vi "Piezo Message Loop.vi"(8 "error in (no error)":errorcluster, 10 "Data Notifiers":T1, 11 "Message Queues":T2) -> (0 "error out":errorcluster)   [LabVIEW 2013, in "Piezo.lvlib"]
uses:
  Piezo.lvlib
  support/Message Queue/All Message Queues.ctl
  support/Message Queue/Message Cluster.ctl
  support/Data Notifiers/All Data Notifiers.ctl
  Acquisition/APD Notifier Cluster.ctl
  Piezo display.ctl
  XY/XY Display.ctl
  Capacitive/Capacitive Signal Cluster.ctl
  Feedback/Error Signal.ctl
  Piezo State.ctl
  Untitled Project 3 Andrea/piezo new/Hardware Configuration Piezo out.ctl
  support/Message Queue/Enqueue Message (Single).vi
  <vilib>/Utility/error.llb/Error Cluster From Error Code.vi
  <vilib>/ErrorRing/Error Ring.xnode
  support/Message Queue/Message Queue.lvlib
  Acquisition/Acquisition.lvlib
  XY/XY.lvlib
  support/Data Notifiers/Data Notifiers.lvlib
  Capacitive/Capacitive.lvlib
  Feedback/Feedback.lvlib
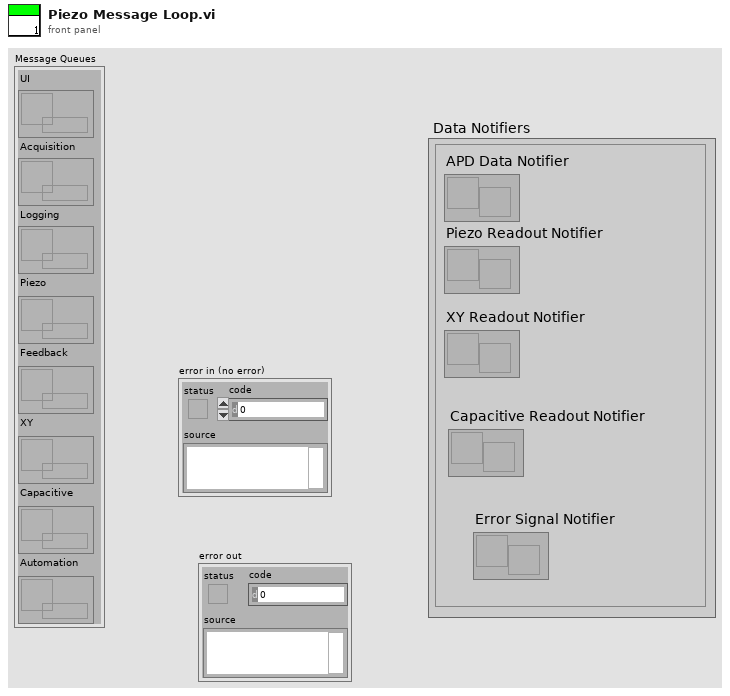
[diagram p1: front panel]
types:
  T1 = typedef "Data Notifiers.lvlib/All Data Notifiers.ctl" = cluster{"APD Data Notifier":refnum<notifier>, "Piezo Readout Notifier":refnum<notifier>, "XY Readout Notifier":refnum<notifier>, "Capacitive Readout Notifier":refnum<notifier>, "Error Signal Notifier":refnum<notifier>}
  T2 = typedef "Message Queue.lvlib/All Message Queues.ctl" = cluster{"UI":refnum<queue>, "Acquisition":refnum<queue>, "Logging":refnum<queue>, "Piezo":refnum<queue>, "Feedback":refnum<queue>, "XY":refnum<queue>, "Capacitive":refnum<queue>, "Automation":refnum<queue>}
  T3 = typedef "Hardware Configuration Piezo out.ctl" = cluster{"physical channels":tag, "MAX   VOLTAGE":dbl, "MIN   VOLTAGE":dbl}
  T4 = typedef "Piezo.lvlib/Piezo State.ctl" = enum16{"Idle", "Acquiring"}
  T5 = typedef "Acquisition.lvlib/APD Notifier Cluster.ctl" = cluster{"data":dbl[][], "t0":i32}
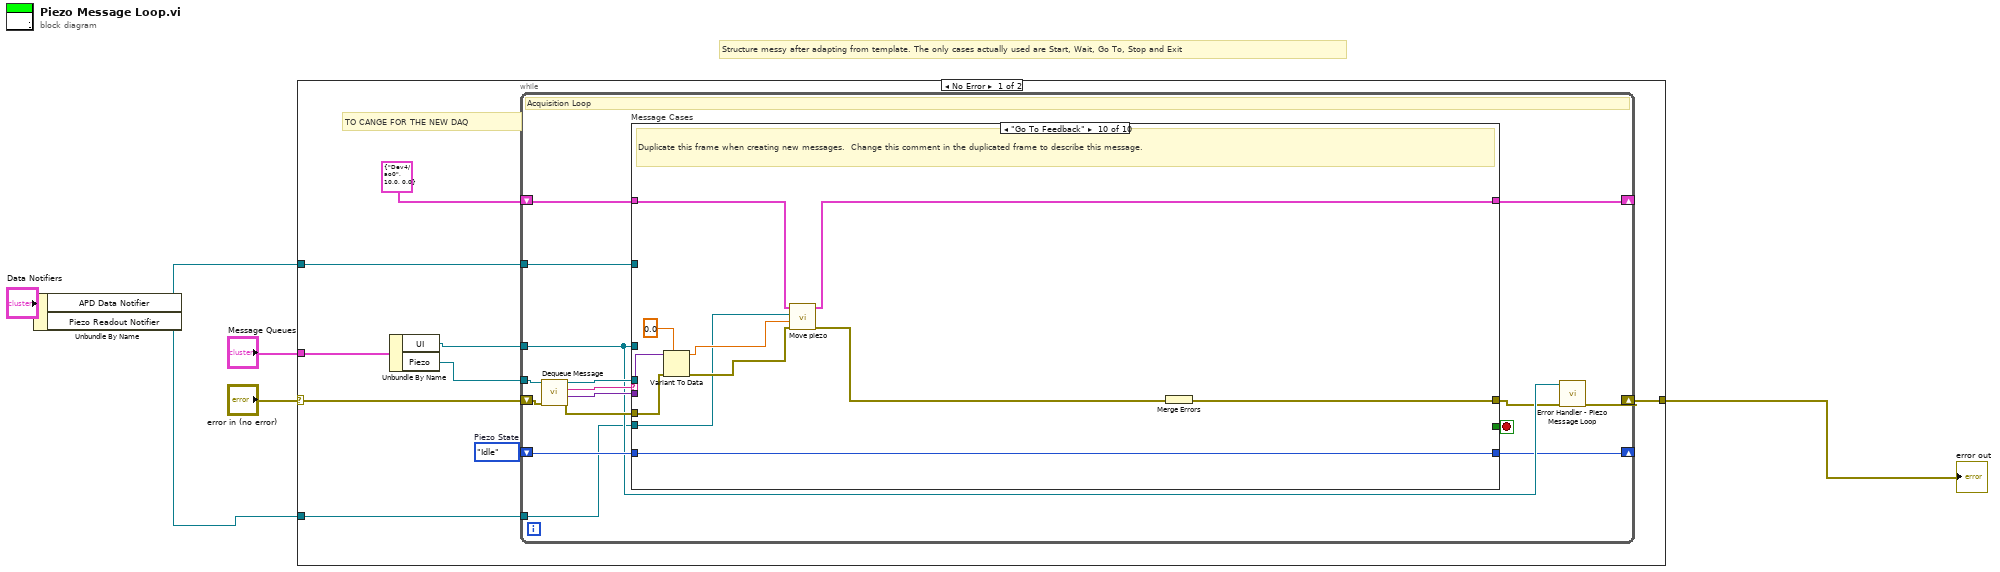
[diagram p0: block diagram]
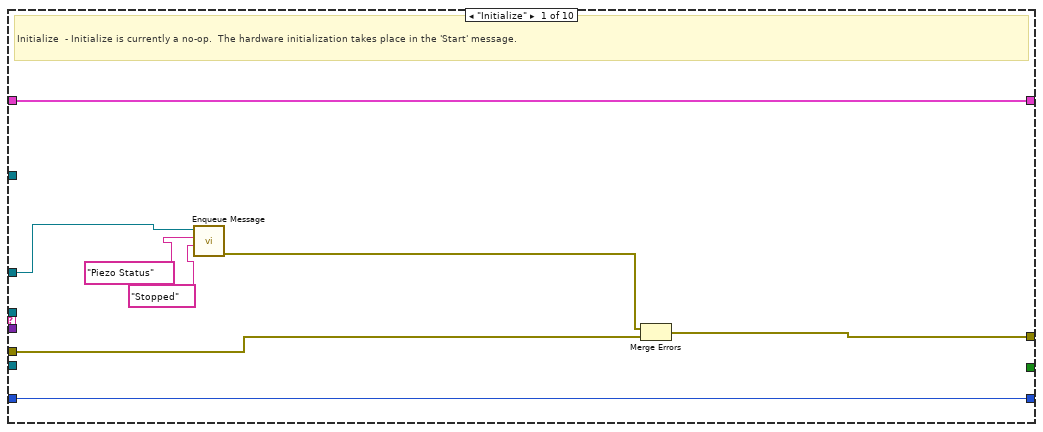
[diagram p2: hidden frame]
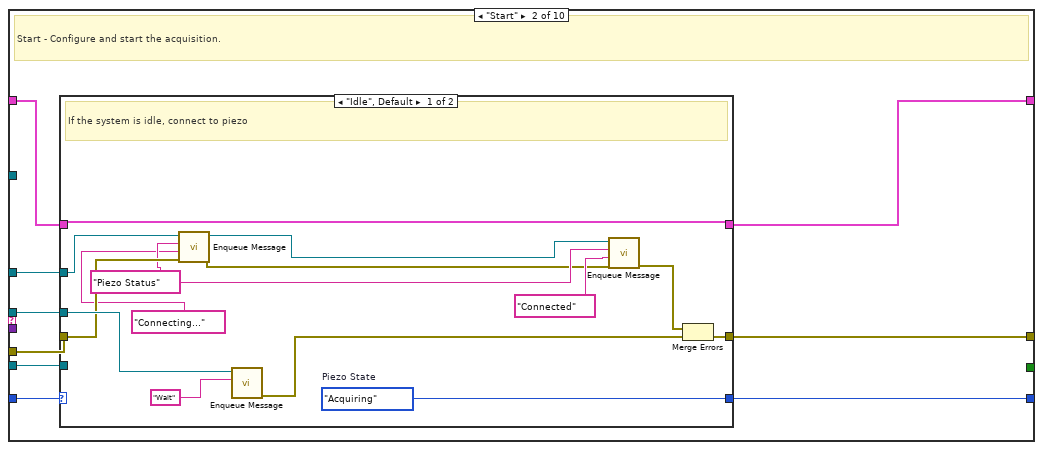
[diagram p3: hidden frame]
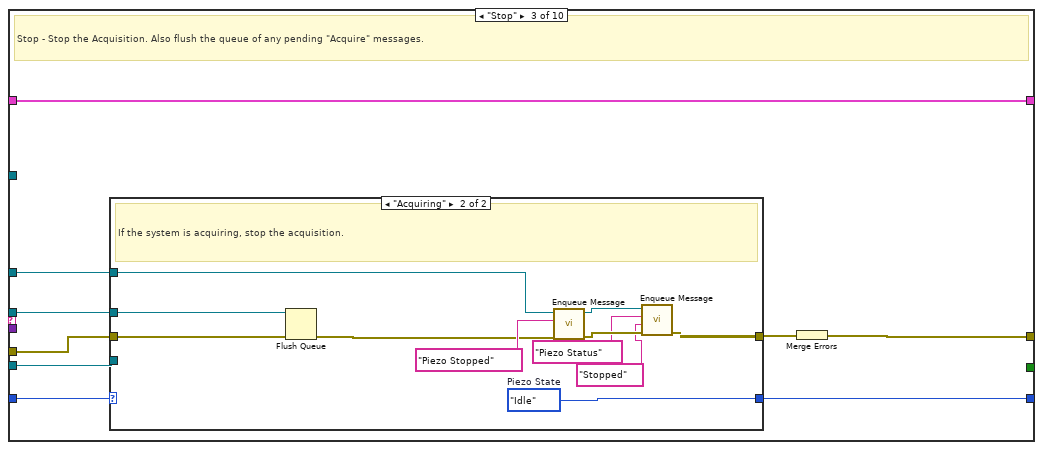
[diagram p5: hidden frame]
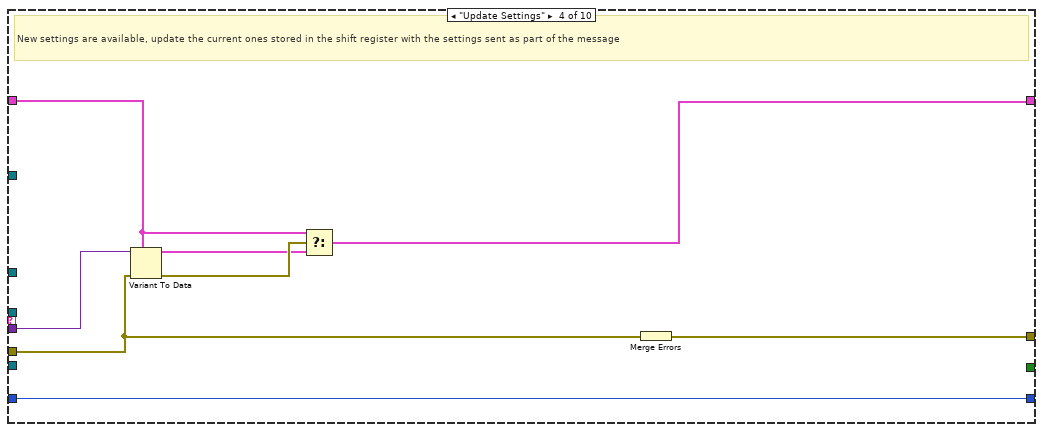
[diagram p7: hidden frame]
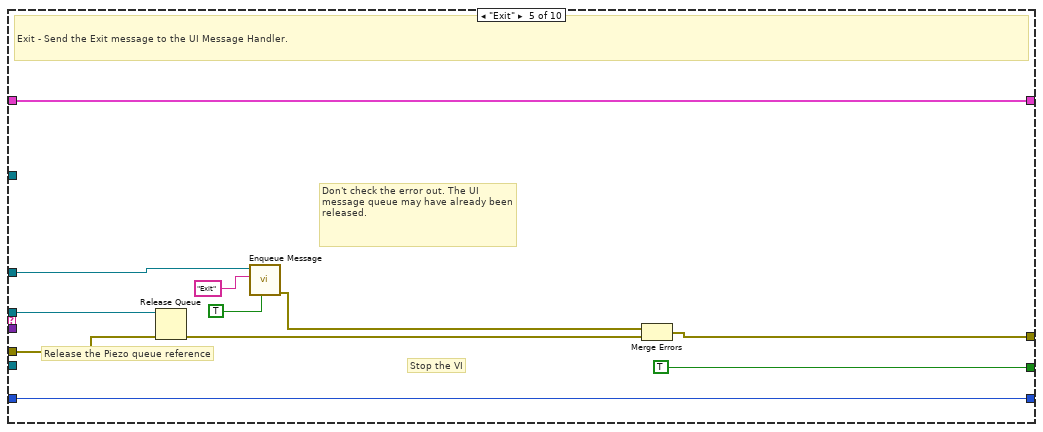
[diagram p8: hidden frame]
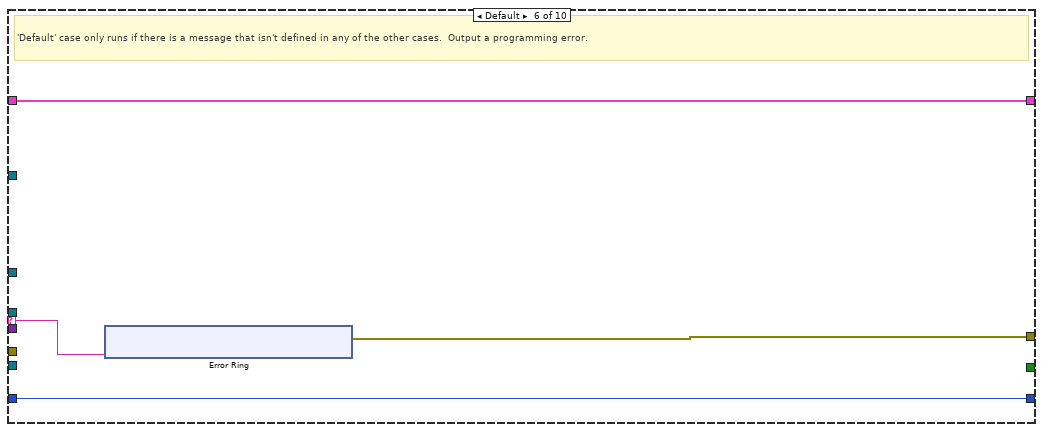
[diagram p9: hidden frame]
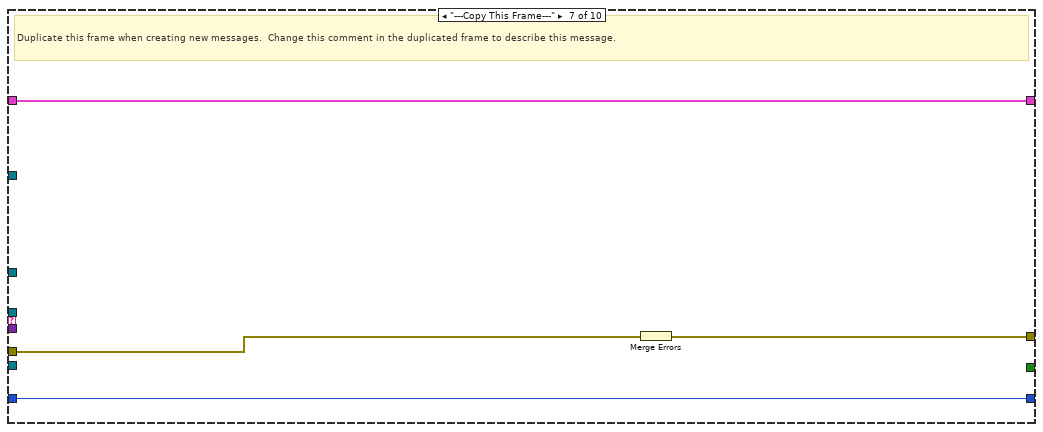
[diagram p10: hidden frame]
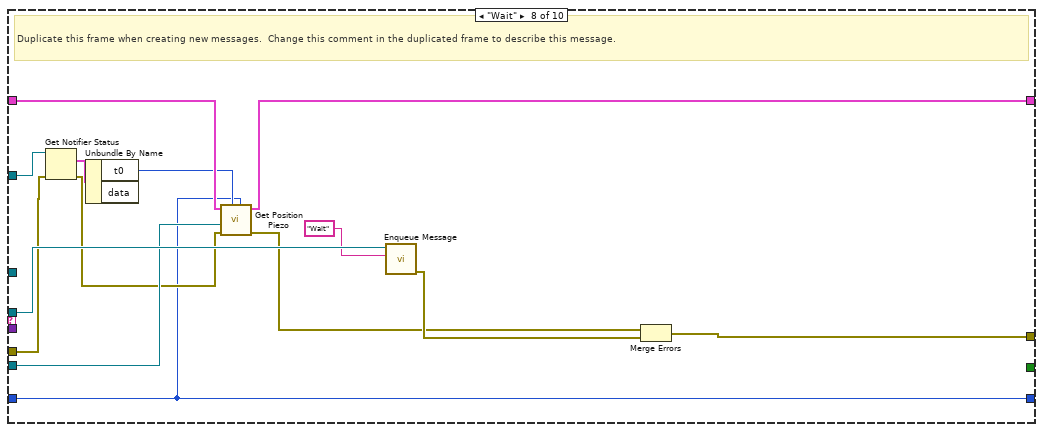
[diagram p11: hidden frame]
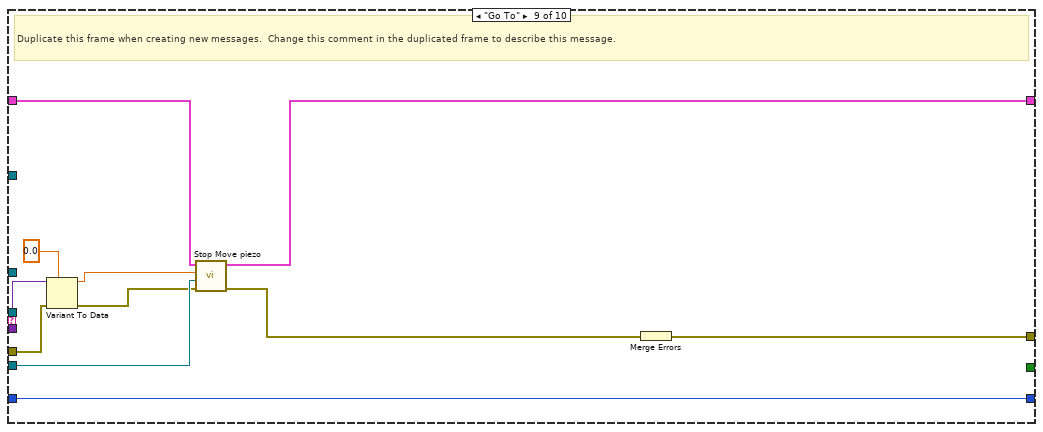
[diagram p12: hidden frame]
diagram:
  # "Structure messy after adapting from template. The only cases actually used are Start, Wait, Go To, Stop and Exit"
  n1 = Unbundle By Name("Data Notifiers") -> ("APD Data Notifier"=w2:refnum<notifier>, "Piezo Readout Notifier"=w1:refnum<notifier>)
  n2 = case shown="No Error" "error in (no error)" {
    selector: "error in (no error)" -> [w10 w158]
    tunnel: "Message Queues" -> [w15 _]
    tunnel: [w13 w158] -> w5
    tunnel: w1 -> [w9 _]
    tunnel: w2 -> [w8 _]
    frame No Error {
      w11 = Piezo_State."Idle"  # Piezo State
      # "TO CANGE FOR THE NEW DAQ"
      n3 = Unbundle By Name(w15) -> ("UI"=w12:refnum<queue>, "Piezo"=w14:refnum<queue>)
      n4 = while {
        tunnel: w14 -> [w24]
        shift-right: [w19] -> _
        shift-left: T3 {"physical channels"="Dev4/ao0", "MAX   VOLTAGE"=10.0, "MIN   VOLTAGE"=0.0} ("Cluster") -> [w31]
        shift-right: [w21] -> w13
        shift-left: w10 -> [w29]
        tunnel: w12 -> [w22]
        shift-right: [w20] -> _
        shift-left: w11 -> [w23]
        tunnel: w9 -> [w17]
        tunnel: w8 -> [w16]
        stop <- w30 stop-if-true
        # "Acquisition Loop"
        n5 = call "Dequeue Message.vi"("error in (no error)"=w29, "Message Queue"=w24) -> ("error out"=w28:errorcluster, "Message Data"=w26:variant, "Message"=w27:string, "dup Message Queue"=w25:refnum<queue>)  [unwired: 6 in]
        n6 = case "Message Cases" shown="\"Go To Feedback\"" w27 {
          selector: w27 -> [_ _ _ _ _ w110 _ _ _ _]
          tunnel: w25 -> [_ w45 w72 _ w102 _ _ w134 _ _]
          tunnel: w28 -> [w38 w46 w73 w90 w104 _ w121 w131 w142 w153]
          tunnel: [w39 w48 w74 w95 w105 w109 w120 w135 w146 w157] -> w18
          tunnel: w31 -> [w36 w47 w67 w91 w96 w107 w118 w128 w141 w147]
          tunnel: [_ _ _ _ TRUE _ _ _ _ _] -> w30
          tunnel: w26 -> [_ _ _ w94 _ _ _ _ w144 w155]
          tunnel: w22 -> [w34 w41 w71 _ w98 _ _ _ _ _]
          tunnel: w23 -> [w37 w44 w70 w89 w101 w108 w119 w123 w145 w156]
          tunnel: [w37 w43 w69 w89 w101 w108 w119 w123 w145 w156] -> w20
          tunnel: [w36 w42 w67 w88 w96 w107 w118 w127 w136 w152] -> w19
          tunnel: w17 -> [_ w40 w66 _ _ _ _ w126 w139 w148]
          tunnel: w16 -> [_ _ _ _ _ _ _ w130 _ _]
          frame "Initialize" {
            # "Initialize  - Initialize is currently a no-op.  The hardware initialization takes place in the 'Start' message."
            n7 = call-poly "Enqueue Message.vi"("Message Data"="Stopped" ("Message"), "Message"="Piezo Status", "Message Queue"=w34) -> ("error out"=w33:errorcluster)  [unwired: 7 in, 1 out]
            n8 = Merge Errors(w33, w38) -> (w39:errorcluster)
          }
          frame "Start" {
            # "Start - Configure and start the acquisition."
            n9 = case shown="\"Idle\", Default" w44 {
              selector: w44 -> [_ w63]
              tunnel: [w62 w65] -> w48
              tunnel: w47 -> [w50 w64]
              tunnel: w46 -> [w54 w65]
              tunnel: w45 -> [w59 _]
              tunnel: [w50 w64] -> w42
              tunnel: [w61 w63] -> w43
              tunnel: w41 -> [w55 _]
              tunnel: w40 -> [_ _]
              frame "Idle", Default {
                w52 = "Piezo Status" ("Message")
                w61 = Piezo_State."Acquiring"  # Piezo State
                # "If the system is idle, connect to piezo"
                n10 = call-poly "Enqueue Message.vi"("error in (no error)"=w54, "Message Data"="Connecting..." ("Message"), "Message"=w52, "Message Queue"=w55) -> ("error out"=w49:errorcluster, "dup Message Queue"=w53:refnum<queue>)  [unwired: 6 in]
                n11 = call-poly "Enqueue Message.vi"("Message"="Wait", "Message Queue"=w59) -> ("error out"=w58:errorcluster)  [unwired: 8 in, 1 out]
                n12 = call-poly "Enqueue Message.vi"("error in (no error)"=w49, "Message Data"="Connected" ("Message"), "Message"=w52, "Message Queue"=w53) -> ("error out"=w57:errorcluster)  [unwired: 6 in, 1 out]
                n13 = Merge Errors(w57, w58) -> (w62:errorcluster)
              }
              frame "Acquiring" {
                # "The system is already acquiring. Ignore the \"Start\" message."
              }
            }
          }
          frame "Stop" {
            # "Stop - Stop the Acquisition. Also flush the queue of any pending \"Acquire\" messages."
            n14 = case shown="\"Acquiring\"" w70 {
              selector: w70 -> [w76 _]
              tunnel: w73 -> [w75 w78]
              tunnel: w72 -> [_ w87]
              tunnel: w71 -> [_ w86]
              tunnel: [w76 w84] -> w69
              tunnel: [w75 w81] -> w68
              tunnel: w66 -> [_ _]
              frame "Idle", Default {
                # "The system is already idle. Ignore the \"Stop\" message."
              }
              frame "Acquiring" {
                w84 = Piezo_State."Idle"  # Piezo State
                # "If the system is acquiring, stop the acquisition."
                n15 = Flush Queue(queue=w87, error in (no error)=w78) -> (error out=w77:errorcluster)  [unwired: 2 out]
                n16 = call-poly "Enqueue Message.vi"("error in (no error)"=w77, "Message"="Piezo Stopped", "Message Queue"=w86) -> ("error out"=w82:errorcluster, "dup Message Queue"=w83:refnum<queue>)  [unwired: 7 in]
                n17 = call-poly "Enqueue Message.vi"("error in (no error)"=w82, "Message Data"="Stopped" ("Message"), "Message"="Piezo Status", "Message Queue"=w83) -> ("error out"=w81:errorcluster)  [unwired: 6 in, 1 out]
              }
            }
            n18 = Merge Errors(w68) -> (w74:errorcluster)
          }
          frame "Update Settings" {
            # "New settings are available, update the current ones stored in the shift register with the settings sent as part of the message"
            n19 = Variant To Data(error in=w90, type=w91, Variant=w94) -> (data=w92:T3, error out=w93:errorcluster)
            n20 = Select(t=w91, s=w93, f=w92) -> (s? t:f=w88:T3)
            n21 = Merge Errors(w90) -> (w95:errorcluster)
          }
          frame "Exit" {
            # "Don't check the error out. The UI message queue may have already been released."
            # "Release the Piezo queue reference"
            # "Stop the VI"
            # "Exit - Send the Exit message to the UI Message Handler."
            n22 = Release Queue(queue=w102, error in (no error)=w104) -> (error out=w103:errorcluster)  [unwired: 1 in, 2 out]
            n23 = call-poly "Enqueue Message.vi"("Priority Message? (F)"=TRUE, "Message"="Exit", "Message Queue"=w98) -> ("error out"=w97:errorcluster)  [unwired: 7 in, 1 out]
            n24 = Merge Errors(w97, w103) -> (w105:errorcluster)
          }
          frame Default {
            # "'Default' case only runs if there is a message that isn't defined in any of the other cases.  Output a programming error."
            n25 = xnode "Error Ring"("parameter 0"=w110) -> ("error out"=w109:errorcluster)
          }
          frame "---Copy This Frame---" {
            # "Duplicate this frame when creating new messages.  Change this comment in the duplicated frame to describe this message."
            n26 = Merge Errors(w121) -> (w120:errorcluster)
          }
          frame "Wait" {
            # "Duplicate this frame when creating new messages.  Change this comment in the duplicated frame to describe this message."
            n27 = Get Notifier Status(notifier=w130, error in (no error)=w131) -> (current notification=w129:T5, error out=w125:errorcluster)  [unwired: 3 out]
            n28 = Unbundle By Name(w129) -> ("t0"=w124:i32)  [unwired: 1 out]
            n29 = call "Get Position Piezo.vi"("Piezo State"=w123, "Counter Time"=w124, "error in (no error)"=w125, "notifier out"=w126, "Cluster"=w128) -> ("error out"=w122:errorcluster, "Cluster 2"=w127:T3)  [unwired: 5 in]
            n30 = call-poly "Enqueue Message.vi"("Message"="Wait", "Message Queue"=w134) -> ("error out"=w132:errorcluster)  [unwired: 8 in, 1 out]
            n31 = Merge Errors(w122, w132) -> (w135:errorcluster)
          }
          frame "Go To" {
            # "Duplicate this frame when creating new messages.  Change this comment in the duplicated frame to describe this message."
            n32 = Variant To Data(error in=w142, type=sgl 0.0, Variant=w144) -> (data=w140:sgl, error out=w138:errorcluster)
            n33 = call "Stop Move piezo.vi"("error in (no error)"=w138, "notifier out"=w139, "MOVE TO [MICRON]"=w140, "Cluster"=w141) -> ("error out"=w137:errorcluster, "Cluster 2"=w136:T3)  [unwired: 6 in]
            n34 = Merge Errors(w137) -> (w146:errorcluster)
          }
          frame "Go To Feedback" {
            # "Duplicate this frame when creating new messages.  Change this comment in the duplicated frame to describe this message."
            n35 = Variant To Data(error in=w153, type=sgl 0.0, Variant=w155) -> (data=w149:sgl, error out=w150:errorcluster)
            n36 = call "Move piezo.vi"("error in (no error)"=w150, "MOVE TO [MICRON]"=w149, "notifier out"=w148, "Hardware Config In"=w147) -> ("error out"=w151:errorcluster, "Hardware Config Out"=w152:T3)  [unwired: 5 in]
            n37 = Merge Errors(w151) -> (w157:errorcluster)
          }
        }
        n38 = call "Error Handler - Piezo Message Loop.vi"("error in (no error)"=w18, "Message Queue"=w22) -> ("dup error in"=w21:errorcluster)  [unwired: 8 in, 1 out]
      }
    }
    frame Error {
    }
  }
  "error out" <- w5
